vi "Joystick_Dell.vi"(8 "Left Analog":dbl, 11 "Right Analog":dbl) -> (0 "Right Motor":dbl, 3 "Left Motor":dbl)   [LabVIEW 2013]
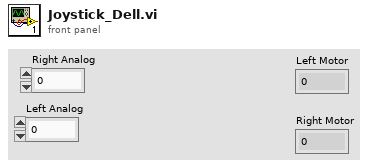
[diagram p1: front panel]
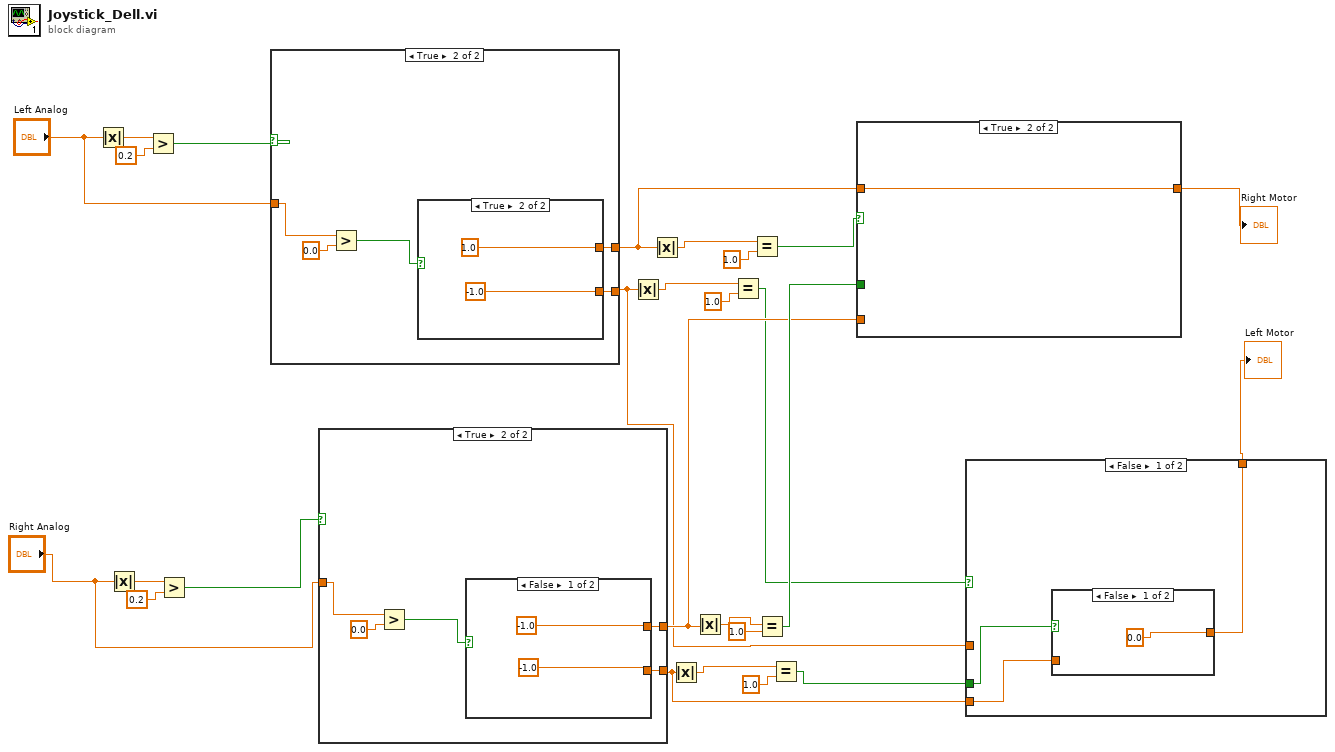
[diagram p0: block diagram]
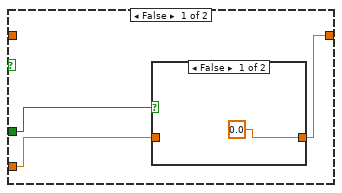
[diagram p4: hidden frame]
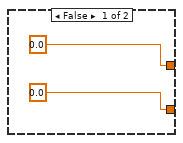
[diagram p6: hidden frame]
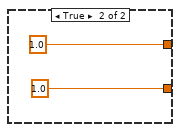
[diagram p7: hidden frame]
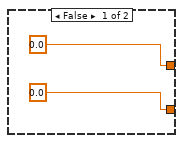
[diagram p8: hidden frame]
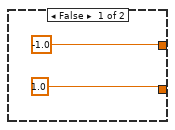
[diagram p9: hidden frame]
diagram:
  n1 = Absolute Value(x="Left Analog") -> (abs(x)=w25:dbl)
  n2 = Absolute Value(x="Right Analog") -> (abs(x)=w21:dbl)
  n3 = Greater?(x=w25, y=0.2) -> (0:w24:bool)
  n4 = Greater?(x=w21, y=0.2) -> (0:w20:bool)
  n5 = case shown="True" w24 {
    tunnel: "Left Analog" -> [_ w33]
    tunnel: [0.0 w30] -> w13
    tunnel: [0.0 w29] -> w4
    frame False {
    }
    frame True {
      n6 = Greater?(x=w33, y=0.0) -> (0:w31:bool)
      n7 = case shown="True" w31 {
        tunnel: [-1.0 1.0] -> w30
        tunnel: [1.0 -1.0] -> w29
        frame False {
        }
        frame True {
        }
      }
    }
  }
  n8 = case shown="True" w20 {
    tunnel: "Right Analog" -> [_ w44]
    tunnel: [0.0 w41] -> w10
    tunnel: [0.0 w40] -> w1
    frame False {
    }
    frame True {
      n9 = Greater?(x=w44, y=0.0) -> (0:w42:bool)
      n10 = case shown="False" w42 {
        tunnel: [-1.0 1.0] -> w41
        tunnel: [-1.0 1.0] -> w40
        frame False {
        }
        frame True {
        }
      }
    }
  }
  n11 = Absolute Value(x=w4) -> (abs(x)=w7:dbl)
  n12 = Absolute Value(x=w13) -> (abs(x)=w18:dbl)
  n13 = Absolute Value(x=w1) -> (abs(x)=w9:dbl)
  n14 = Absolute Value(x=w10) -> (abs(x)=w15:dbl)
  n15 = Equal?(x=w7, y=1.0) -> (x = y?=w5:bool)
  n16 = Equal?(x=w18, y=1.0) -> (x = y?=w14:bool)
  n17 = Equal?(x=w15, y=1.0) -> (x = y?=w11:bool)
  n18 = Equal?(x=w9, y=1.0) -> (x = y?=w2:bool)
  n19 = case shown="True" w14 {
    tunnel: w13 -> [_ w54]
    tunnel: [w49 w54] -> w12
    tunnel: w11 -> [w51 _]
    tunnel: w10 -> [w50 _]
    frame False {
      n20 = case shown="False" w51 {
        tunnel: w50 -> [_ w53]
        tunnel: [0.0 w53] -> w49
        frame False {
        }
        frame True {
        }
      }
    }
    frame True {
    }
  }
  "Right Motor" <- w12
  n21 = case shown="False" w5 {
    tunnel: w4 -> [_ w60]
    tunnel: [w55 w60] -> w3
    tunnel: w2 -> [w57 _]
    tunnel: w1 -> [w56 _]
    frame False {
      n22 = case shown="False" w57 {
        tunnel: w56 -> [_ w59]
        tunnel: [0.0 w59] -> w55
        frame False {
        }
        frame True {
        }
      }
    }
    frame True {
    }
  }
  "Left Motor" <- w3
